vi "Mode Matrix Name SLM.vi"   [LabVIEW 2014]
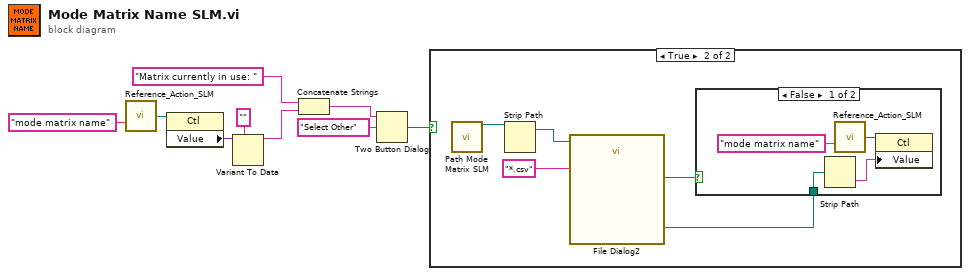
[diagram p0: block diagram]
diagram:
  n1 = call "Reference_Action_SLM.vi"("Control Name"="mode matrix name") -> ("Ref OUT"=w4:refnum<vi>)  [unwired: 12 in, 2 out]
  n2 = property class="Ctl"(reference=w4) -> ("Value"=w5:variant)  [unwired: 1 in, 2 out]
  n3 = Variant To Data(type="" ("string"), Variant=w5) -> (data=w1:string)  [unwired: 1 in, 1 out]
  n4 = Concatenate Strings("Matrix currently in use: " ("string"), w1) -> (w8:string)
  n5 = Two Button Dialog(message=w8, 2:"Select Other" ("T button name (\"OK\")")) -> (T button?=w6:bool)  [unwired: 1 out]
  n6 = case shown="True" w6 {
    frame False {
    }
    frame True {
      n7 = call "Path Mode Matrix SLM.vi"() -> ("mode matrix path"=w11:path)  [unwired: 15 in]
      n8 = Strip Path(path=w11) -> (stripped path=w10:path)  [unwired: 1 out]
      n9 = call "File Dialog2"("start path"=w10, "pattern (all files)"="*.csv" ("string")) -> ("selected path"=w12:path, "cancelled"=w13:bool)  [unwired: 5 in, 7 out]
      n10 = case shown="False" w13 {
        tunnel: w12 -> [w16 _]
        frame False {
          n11 = Strip Path(path=w16) -> (name=w15:string)  [unwired: 1 out]
          n12 = call "Reference_Action_SLM.vi"("Control Name"="mode matrix name") -> ("Ref OUT"=w18:refnum<vi>)  [unwired: 12 in, 2 out]
          n13 = property class="Ctl"(reference=w18, "Value"=w15) -> ()  [unwired: 1 in, 2 out]
        }
        frame True {
        }
      }
    }
  }
